vi "process_result.vi"(2 "reference 2":refnum<vi>, 3 "reuslt cmd":string[](array[string])) -> ()   [LabVIEW 2026]
uses:
  <vilib>/Utility/miscctls.llb/LVRowAndColumnTypeDef.ctl
panel:
  in  "Multicolumn Listbox":i32(listbox)
  out "result table output":i32(listbox)
  in  "result table intput":i32(listbox)
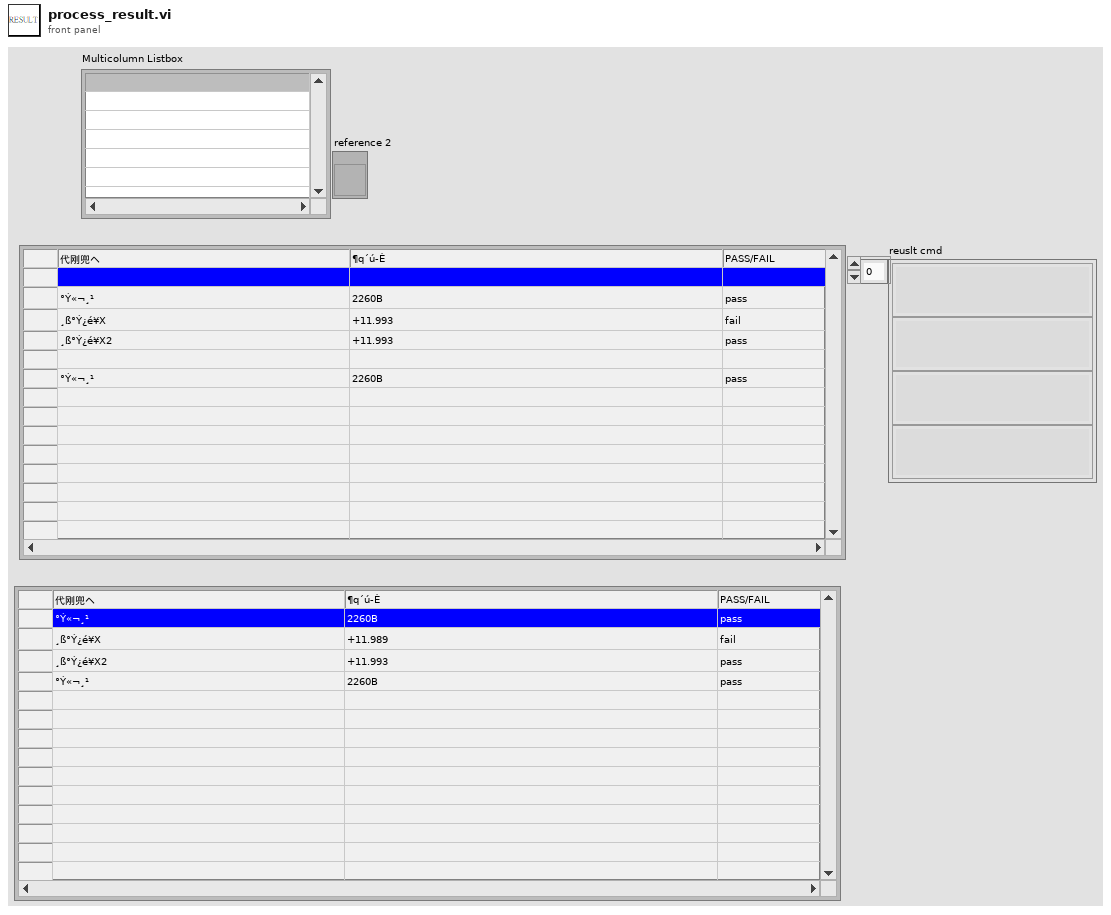
[diagram p1: front panel]
types:
  T1 = typedef "LVRowAndColumnTypeDef.ctl" = cluster{"Row":i32, "Column":i32}
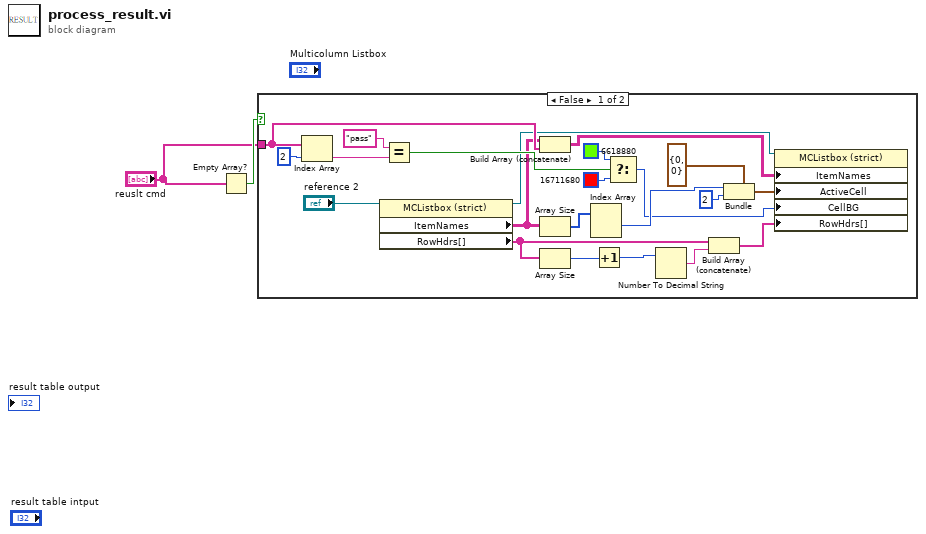
[diagram p0: block diagram]
diagram:
  n1 = Empty Array?(array="reuslt cmd") -> (empty?=w2:bool)
  n2 = case shown="False" w2 {
    tunnel: "reuslt cmd" -> [w11 _]
    frame False {
      n3 = Index Array(array=w11, index=2) -> (element=w23:string)
      n4 = property class="MCListbox (strict)"(reference="reference 2") -> (reference out=w10:refnum<vi>, "ItemNames"=w9:string[][], "RowHdrs[]"=w3:string[])  [unwired: 1 in, 1 out]
      n5 = Equal?(x="pass", y=w23) -> (x = y?=w24:bool)
      n6 = Build Array (concatenate)(w9, w11) -> (w14:string[][])
      n7 = Array Size(array=w9) -> (size(s)=w21:i32[])
      n8 = Array Size(array=w3) -> (size(s)=w7:i32)
      n9 = Index Array(array=w21) -> (element #1=w22:i32)  [unwired: 2 in, 1 out]
      n10 = Increment(x=w7) -> (x+1=w6:i32)
      n11 = Select(t=u32 6618880 ("Active Cell:Cell Background Color"), s=w24, f=u32 16711680 ("Active Cell:Cell Background Color")) -> (s? t:f=w12:u32)
      n12 = Number To Decimal String(number=w6) -> (decimal integer string=w5:string)  [unwired: 1 in]
      n13 = Build Array (concatenate)(w3, w5) -> (w4:string[])
      n14 = Bundle(cluster=T1 {"Row"=0, "Column"=0} ("Active Cell:Active Cell"), "Row"=w22, "Column"=2 ("Row")) -> (w13:T1)
      n15 = property class="MCListbox (strict)"(reference=w10, "ItemNames"=w14, "ActiveCell"=w13, "CellBG"=w12, "RowHdrs[]"=w4) -> ()  [unwired: 1 in, 2 out]
    }
    frame True {
    }
  }
